vi "FPGA VI_Multiple Groups_Multiple Rates_Simulated_WithNoise_Example.vi"() -> ()   [LabVIEW 2019]
uses:
  <vilib>/rvi/DataTransferAndStorage/Container/XNode/niFpgaContainer.xnode
  <vilib>/Platform/TimedLoop/XDataNode/XDataNode.xnode
  <vilib>/Platform/TimedLoop/XDataNode/nitl_modes.ctl
  <vilib>/Platform/TimedLoop/XDataNode/XDNodeRunTimeDep.lvlib
  <vilib>/Platform/TimedLoop/XDataNode/wakeup.ctl
  <vilib>/Platform/TimedLoop/XDataNode/timing_clust.ctl
  <vilib>/rvi/FIFO/Fifo_Resource/niFpgaFifoEmulationRefIn.vi
  Types/Injection.Core.Internal.Settings.ctl
  <vilib>/rvi/LocalResourceManager/LocalResourceManager.xnode
  <vilib>/rvi/DataTransferAndStorage/Container/Common/niFpgaContainerGetUniqueNameForEmu.vi
  <vilib>/rvi/DataTransferAndStorage/Container/Common/niFpgaContainerSetEmuInfo.vi
  <vilib>/rvi/eio/common/nirviEmuReportErrorAndStop.vi
  <vilib>/rvi/Memory/Memory_Emulation/nirvimemoryFastEmulation.vi
  <vilib>/rvi/Memory/Memory_Emulation/nirvimemoryEmulation.vi
  Types/Injection.Mux.State.ctl
  <vilib>/rvi/interface/RandomDataEmulation/nirviRandomDataFpgaReadWriteTemplate.vi
  Types/Injection.Timing.ctl
  Types/Injection.Core.Settings.ctl
  Types/Injection.Global.Settings.ctl
panel:
  out "Intermediate FIFO Write Timeout 2":bool
  in  "Settings.Global.DUT1":T1={"Enable?"=FALSE, "Initial Voltage Threshold"=12.0, "Event Dwell Limit"=2000, "Voltage Gain"=1.0, "Current Gain"=1.0, "Filter Samples"=5, "Pretrigger Samples"=5, "Active Edge"=TRUE}
  in  "Settings.Index0.DUT1.Injector0":T2
  in  "Settings.Index1.DUT1.Injector1":T2
  in  "Settings.Index2.DUT1.Injector2":T2
  in  "Settings.Index3.DUT1.Injector3":T2
  out "Acqusition Loop Ticks 2":u32
  in  "Settings.Timing.DUT1":T3={"Injection Sample Period (Ticks)"=80}
  in  "Settings.Global.DUT2":T1={"Enable?"=FALSE, "Initial Voltage Threshold"=12.0, "Event Dwell Limit"=2000, "Voltage Gain"=1.0, "Current Gain"=1.0, "Filter Samples"=5, "Pretrigger Samples"=5, "Active Edge"=TRUE}
  in  "Settings.Index6.DUT2.Injector2":T2
  in  "Settings.Index7.DUT2.Injector3":T2
  out "Intermediate FIFO Write Timeout":bool
  in  "Settings.Index4.DUT2.Injector0":T2
  in  "Settings.Index5.DUT2.Injector1":T2
  in  "Settings.Timing.DUT2":T3={"Injection Sample Period (Ticks)"=320}
  out "Acqusition Loop Ticks":u32
  in  "Settings.DMA":cluster{"# of Injectors":u8}={"# of Injectors"=8}
  out "Host DMA Out?":bool
  out "Intermediate Time Out?":bool
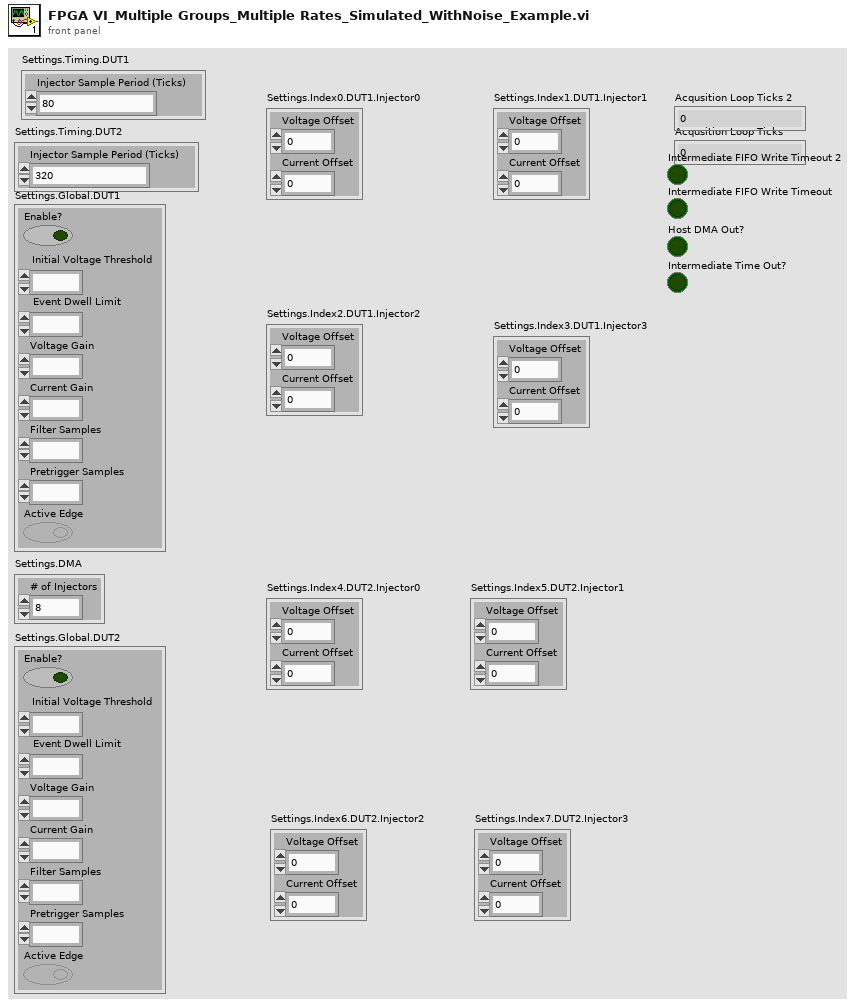
[diagram p1: front panel]
types:
  T1 = typedef "Injection.Global.Settings.ctl" = cluster{"Enable?":bool, "Initial Voltage Threshold":fxp<+/-,32,8>, "Event Dwell Limit":u16, "Voltage Gain":fxp<+/-,32,8>, "Current Gain":fxp<+/-,32,8>, "Filter Samples":u8, "Pretrigger Samples":u8, "Active Edge":bool}
  T2 = typedef "Injection.Core.Settings.ctl" = cluster{"Voltage Offset":fxp<+/-,32,8>, "Current Offset":fxp<+/-,32,8>}
  T3 = typedef "Injection.Timing.ctl" = cluster{"Injection Sample Period (Ticks)":u32}
  T4 = cluster{"Data.Samples":u32, "Injection.Period":u32, "Injector.Index":u8, "Iteration":u32}
  T5 = typedef "Injection.Mux.State.ctl" = enum8{"Wait on Transfer", "Transfer Injector Index", "Transfer # of Samples", "Transfer Injection Period", "Transfer Data Samples"}
  T6 = typedef "Injection.Core.Internal.Settings.ctl" = cluster{"Data Buffer FIFO":refnum<k21>, "Capture Complete Trigger FIFO":refnum<k21>}
  T7 = typedef "XDNodeRunTimeDep.lvlib/timing_clust.ctl" = cluster{"Expected End [f-1]":u64, "Actual End [f-1]":u64, "Finished Late? [f-1]":bool, "Expected End [i-1]":u64, "Actual End [i-1]":u64, "Finished Late? [i-1]":bool, "Expected Start [i]":u64, "Actual Start [i]":u64, "Expected Start [f]":u64, "Actual Start [f]":u64, "Source Name":string, "Structure Name":string, "Period":i64, "Deadline":i64, "Offset":i64, "Start":i64, "Priority":i32, "Timeout":i32, "Mode":T8, "Wakeup Reason":T9, "Error":errorcluster, "Source Type":string, "Secondary Source Type":string, "Global End Time":u64, "Global Start Time":u64, "Frame Duration":u64, "Iteration Duration":u64, "Assigned CPU":i32, "I/O Scan Engine Mode":u32}
  T8 = typedef "XDNodeRunTimeDep.lvlib/nitl_modes.ctl" = enum32{"No Change", "Process missed periods, maintain original phase", "Discard missed periods, maintain original phase", "Process missed periods, ignore original phase", "Discard missed periods, ignore original phase"}
  T9 = typedef "XDNodeRunTimeDep.lvlib/wakeup.ctl" = enum32{"Normal", "Aborted", "Asynchronous wakeup", "Timing source error", "Timed loop error", "Timeout"}
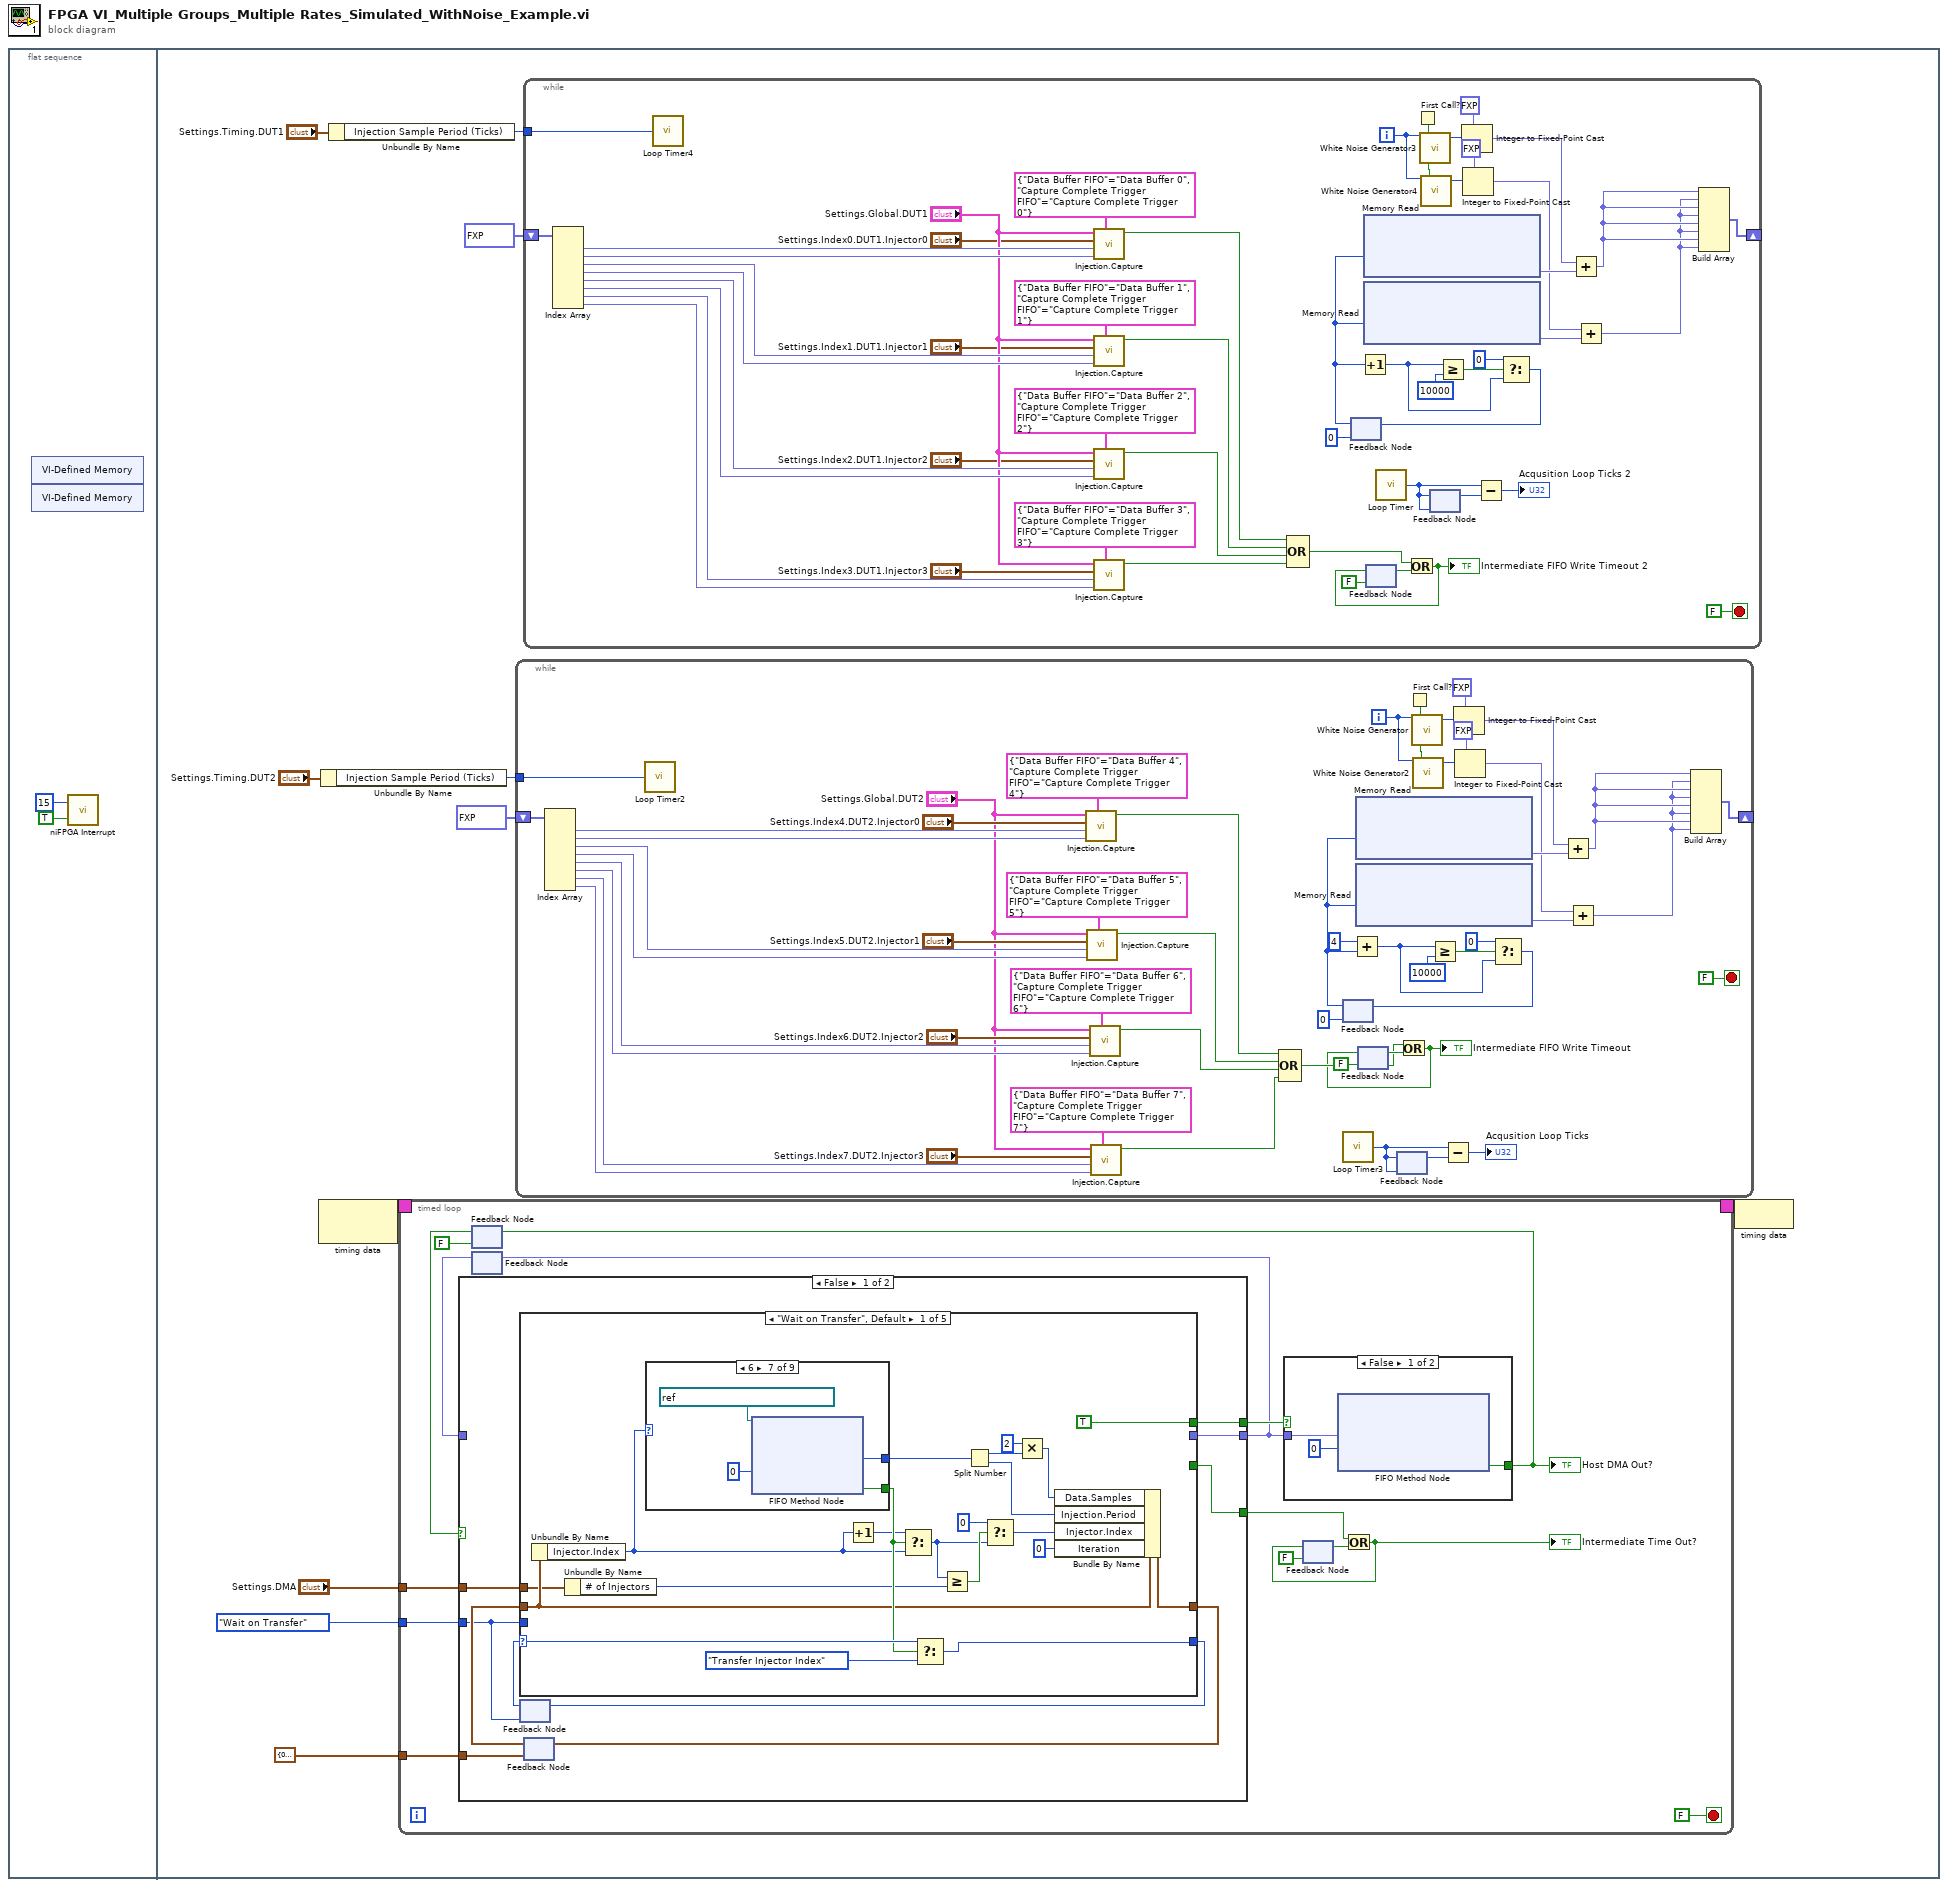
[diagram p0: block diagram]
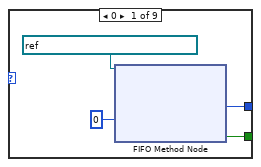
[diagram p2: hidden frame]
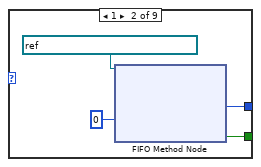
[diagram p3: hidden frame]
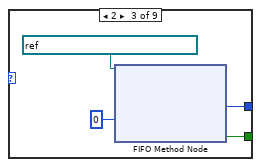
[diagram p4: hidden frame]
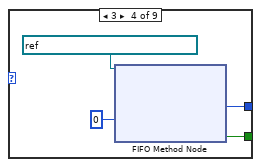
[diagram p5: hidden frame]
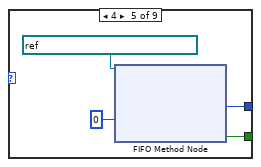
[diagram p6: hidden frame]
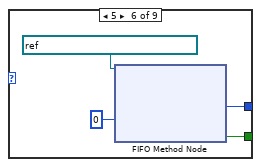
[diagram p7: hidden frame]
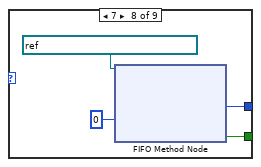
[diagram p8: hidden frame]
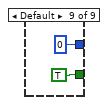
[diagram p9: hidden frame]
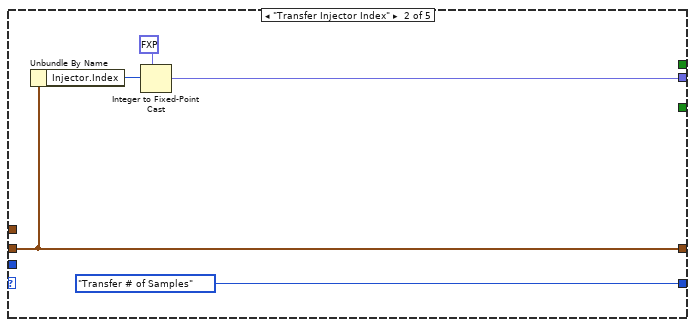
[diagram p10: hidden frame]
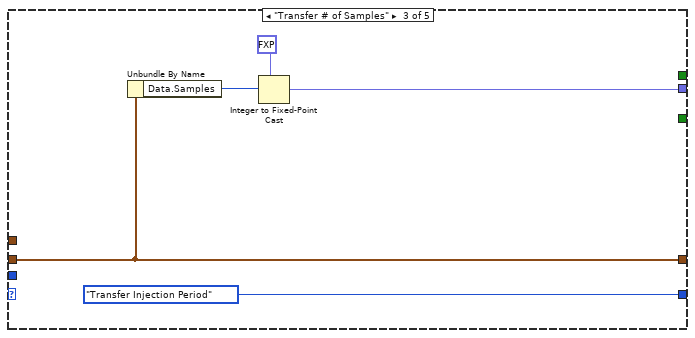
[diagram p11: hidden frame]
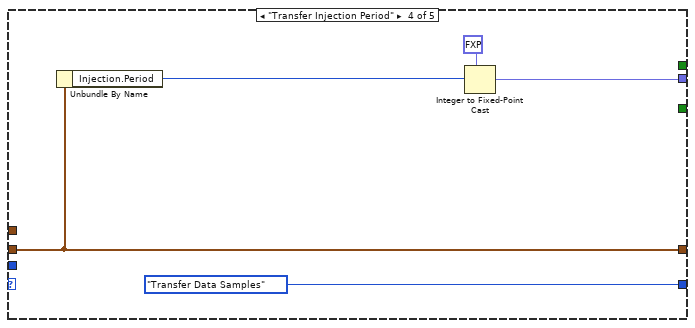
[diagram p12: hidden frame]
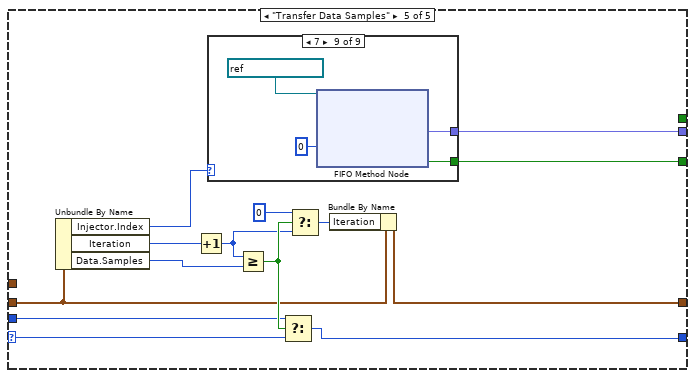
[diagram p13: hidden frame]
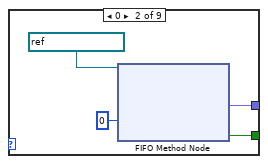
[diagram p15: hidden frame]
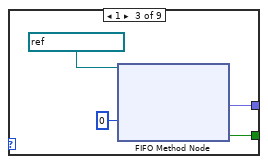
[diagram p16: hidden frame]
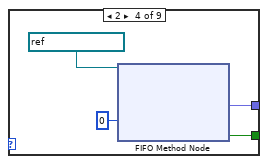
[diagram p17: hidden frame]
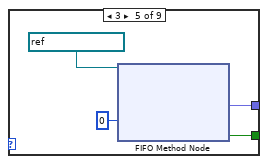
[diagram p18: hidden frame]
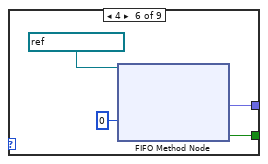
[diagram p19: hidden frame]
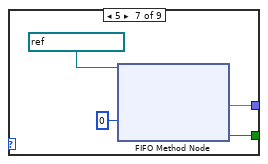
[diagram p20: hidden frame]
diagram:
  n1 = flat-sequence {
    frame #0 {
      n2 = xnode "VI-Defined Memory"() -> ()  [unwired: 1 out]
      n3 = xnode "VI-Defined Memory"() -> ()  [unwired: 1 out]
      n4 = call <vilib>:"niFPGA Interrupt.vi"("Wait Until Cleared (F)"=TRUE, "IRQ Number (0)"=u8 15) -> ()  [unwired: 1 in]
    }
    frame #1 {
      n5 = node-c288() -> (w13:T7)  [unwired: 1 in]
      n6 = Unbundle By Name("Settings.Timing.DUT2") -> ("Injection Sample Period (Ticks)"=w6:u32)
      n7 = Unbundle By Name("Settings.Timing.DUT1") -> ("Injection Sample Period (Ticks)"=w5:u32)
      n8 = timed-loop {
        timing: w13 -> [_]
        timing-out: [_] -> w12
        tunnel: "Settings.DMA" -> [w68]
        tunnel: Injection.Mux.State."Wait on Transfer" -> [w67]
        tunnel: T4 {"Data.Samples"=0, "Injection.Period"=0, "Injector.Index"=0, "Iteration"=0} ("Local.Data") -> [w66]
        stop <- FALSE stop-if-true
        n9 = feedback #1(FALSE ("Timed Out?")) -> (w76:bool)
        n10 = feedback #2() -> (w73:fxp<+/-,32,8>)  [unwired: 1 in]
        n11 = case shown="False" w76 {
          tunnel: [w88 w206] -> w74
          tunnel: [w87 w205] -> w78
          tunnel: w67 -> [w81 _]
          tunnel: [w86 w205] -> w69
          tunnel: w68 -> [w85 _]
          tunnel: w66 -> [w82 _]
          tunnel: w73 -> [_ w206]
          frame False {
            n12 = feedback #3(w81) -> (w80:T5)
            n13 = feedback #4(w82) -> (w83:T4)
            n14 = case shown="\"Wait on Transfer\", Default" w80 {
              selector: w80 -> [w109 _ _ _ w166]
              tunnel: w83 -> [w100 w147 w151 w155 w164]
              tunnel: [w108 w147 w151 w155 w163] -> w84
              tunnel: [w107 Injection.Mux.State."Transfer # of Samples" Injection.Mux.State."Transfer Injection Period" Injection.Mux.State."Transfer Data Samples" w165] -> w79
              tunnel: [_ w146 w150 w157 w162] -> w88
              tunnel: [TRUE _ _ _ _] -> w87
              tunnel: w81 -> [_ _ _ _ w159]
              tunnel: [_ _ _ _ w161] -> w86
              tunnel: w85 -> [w97 _ _ _ _]
              frame "Wait on Transfer", Default {
                n15 = Unbundle By Name(w100) -> ("Injector.Index"=w99:u8)
                n16 = Unbundle By Name(w97) -> ("# of Injectors"=w96:u8)
                n17 = case shown="6" w99 {
                  tunnel: [w112 w116 w120 w124 w128 w132 w136 w140 u64 0 ("Element")] -> w95
                  tunnel: [w111 w115 w119 w123 w127 w131 w135 w139 TRUE ("Timed Out?")] -> w105
                  frame 0 {
                    n18 = xnode ("FIFO Method Node")("Timeout"=0, "FIFO In"=refnum<k21> "Capture Complete Trigger 0") -> ("Element"=w112:u64, "Timed Out?"=w111:bool)  [unwired: 1 out]
                  }
                  frame 1 {
                    n19 = xnode ("FIFO Method Node")("Timeout"=0, "FIFO In"=refnum<k21> "Capture Complete Trigger 1") -> ("Element"=w116:u64, "Timed Out?"=w115:bool)  [unwired: 1 out]
                  }
                  frame 2 {
                    n20 = xnode ("FIFO Method Node")("Timeout"=0, "FIFO In"=refnum<k21> "Capture Complete Trigger 2") -> ("Element"=w120:u64, "Timed Out?"=w119:bool)  [unwired: 1 out]
                  }
                  frame 3 {
                    n21 = xnode ("FIFO Method Node")("Timeout"=0, "FIFO In"=refnum<k21> "Capture Complete Trigger 3") -> ("Element"=w124:u64, "Timed Out?"=w123:bool)  [unwired: 1 out]
                  }
                  frame 4 {
                    n22 = xnode ("FIFO Method Node")("Timeout"=0, "FIFO In"=refnum<k21> "Capture Complete Trigger 4") -> ("Element"=w128:u64, "Timed Out?"=w127:bool)  [unwired: 1 out]
                  }
                  frame 5 {
                    n23 = xnode ("FIFO Method Node")("Timeout"=0, "FIFO In"=refnum<k21> "Capture Complete Trigger 5") -> ("Element"=w132:u64, "Timed Out?"=w131:bool)  [unwired: 1 out]
                  }
                  frame 6 {
                    n24 = xnode ("FIFO Method Node")("Timeout"=0, "FIFO In"=refnum<k21> "Capture Complete Trigger 6") -> ("Element"=w136:u64, "Timed Out?"=w135:bool)  [unwired: 1 out]
                  }
                  frame 7 {
                    n25 = xnode ("FIFO Method Node")("Timeout"=0, "FIFO In"=refnum<k21> "Capture Complete Trigger 7") -> ("Element"=w140:u64, "Timed Out?"=w139:bool)  [unwired: 1 out]
                  }
                  frame Default {
                  }
                }
                n26 = Increment(x=w99) -> (x+1=w104:u8)
                n27 = Select(t=w104, s=w105, f=w99) -> (s? t:f=w102:u8)
                n28 = Select(t=w109, s=w105, f=Injection.Mux.State."Transfer Injector Index") -> (s? t:f=w107:T5)
                n29 = Greater Or Equal?(x=w102, y=w96) -> (x >= y?=w103:bool)
                n30 = Split Number(x=w95) -> (hi(x)=w94:u32, lo(x)=w93:u32)
                n31 = Select(t=u8 0, s=w103, f=w102) -> (s? t:f=w98:u8)
                n32 = Multiply(x=u32 2, y=w94) -> (x*y=w91:u32)
                n33 = Bundle By Name(cluster=w100, "Data.Samples"=w91, "Injection.Period"=w93, "Injector.Index"=w98, "Iteration"=u32 0) -> (w108:T4)
              }
              frame "Transfer Injector Index" {
                n34 = Unbundle By Name(w147) -> ("Injector.Index"=w148:u8)
                n35 = Integer to Fixed-Point Cast(fixed-point type=fxp<+/-,32,8> 0.0, integer=w148) -> (fixed-point=w146:fxp<+/-,32,8>)
              }
              frame "Transfer # of Samples" {
                n36 = Unbundle By Name(w151) -> ("Data.Samples"=w152:u32)
                n37 = Integer to Fixed-Point Cast(fixed-point type=fxp<+/-,32,8> 0.0, integer=w152) -> (fixed-point=w150:fxp<+/-,32,8>)
              }
              frame "Transfer Injection Period" {
                n38 = Unbundle By Name(w155) -> ("Injection.Period"=w156:u32)
                n39 = Integer to Fixed-Point Cast(fixed-point type=fxp<+/-,32,8> 0.0, integer=w156) -> (fixed-point=w157:fxp<+/-,32,8>)
              }
              frame "Transfer Data Samples" {
                n40 = Unbundle By Name(w164) -> ("Injector.Index"=w172:u8, "Iteration"=w167:u32, "Data.Samples"=w160:u32)
                n41 = Increment(x=w167) -> (x+1=w169:u32)
                n42 = case shown="7" w172 {
                  tunnel: [_ w175 w179 w183 w187 w191 w195 w199 w203] -> w162
                  tunnel: [_ w174 w178 w182 w186 w190 w194 w198 w202] -> w161
                  frame Default {
                  }
                  frame 0 {
                    n43 = xnode ("FIFO Method Node")("Timeout"=0, "FIFO In"=refnum<k21> "Data Buffer 0" ("Voltage FIFO")) -> ("Element"=w175:fxp<+/-,32,8>, "Timed Out?"=w174:bool)  [unwired: 1 out]
                  }
                  frame 1 {
                    n44 = xnode ("FIFO Method Node")("Timeout"=0, "FIFO In"=refnum<k21> "Data Buffer 1" ("Voltage FIFO")) -> ("Element"=w179:fxp<+/-,32,8>, "Timed Out?"=w178:bool)  [unwired: 1 out]
                  }
                  frame 2 {
                    n45 = xnode ("FIFO Method Node")("Timeout"=0, "FIFO In"=refnum<k21> "Data Buffer 2" ("Voltage FIFO")) -> ("Element"=w183:fxp<+/-,32,8>, "Timed Out?"=w182:bool)  [unwired: 1 out]
                  }
                  frame 3 {
                    n46 = xnode ("FIFO Method Node")("Timeout"=0, "FIFO In"=refnum<k21> "Data Buffer 3" ("Voltage FIFO")) -> ("Element"=w187:fxp<+/-,32,8>, "Timed Out?"=w186:bool)  [unwired: 1 out]
                  }
                  frame 4 {
                    n47 = xnode ("FIFO Method Node")("Timeout"=0, "FIFO In"=refnum<k21> "Data Buffer 4" ("Voltage FIFO")) -> ("Element"=w191:fxp<+/-,32,8>, "Timed Out?"=w190:bool)  [unwired: 1 out]
                  }
                  frame 5 {
                    n48 = xnode ("FIFO Method Node")("Timeout"=0, "FIFO In"=refnum<k21> "Data Buffer 5" ("Voltage FIFO")) -> ("Element"=w195:fxp<+/-,32,8>, "Timed Out?"=w194:bool)  [unwired: 1 out]
                  }
                  frame 6 {
                    n49 = xnode ("FIFO Method Node")("Timeout"=0, "FIFO In"=refnum<k21> "Data Buffer 6" ("Voltage FIFO")) -> ("Element"=w199:fxp<+/-,32,8>, "Timed Out?"=w198:bool)  [unwired: 1 out]
                  }
                  frame 7 {
                    n50 = xnode ("FIFO Method Node")("Timeout"=0, "FIFO In"=refnum<k21> "Data Buffer 7" ("Voltage FIFO")) -> ("Element"=w203:fxp<+/-,32,8>, "Timed Out?"=w202:bool)  [unwired: 1 out]
                  }
                }
                n51 = Greater Or Equal?(x=w169, y=w160) -> (x >= y?=w171:bool)
                n52 = Select(t=w159, s=w171, f=w166) -> (s? t:f=w165:T5)
                n53 = Select(t=u32 0, s=w171, f=w169) -> (s? t:f=w168:u32)
                n54 = Bundle By Name(cluster=w164, "Iteration"=w168) -> (w163:T4)
              }
            }
            n55 = feedback-in #3(w79) -> ()
            n56 = feedback-in #4(w84) -> ()
          }
          frame True {
            w205 = FALSE
          }
        }
        n57 = feedback-in #2(w74) -> ()
        n58 = case shown="False" w78 {
          tunnel: w74 -> [w208 _]
          tunnel: [w207 FALSE ("Timed Out?")] -> w77
          frame False {
            n59 = xnode ("FIFO Method Node")("Element"=w208, "Timeout"=0) -> ("Timed Out?"=w207:bool)  [unwired: 1 in, 1 out]
          }
          frame True {
          }
        }
        "Host DMA Out?" <- w77
        n60 = feedback-in #1(w77) -> ()
        n61 = feedback #5(FALSE ("Timed Out?")) -> (w71:bool)
        n62 = Or(x=w69, y=w71) -> (x .or. y?=w70:bool)
        "Intermediate Time Out?" <- w70
        n63 = feedback-in #5(w70) -> ()
      }
      n64 = while {
        shift-right: [w238] -> _
        shift-left: fxp<+/-,24,5>[] [0.0, 0.0, 0.0, 0.0, 0.0, 0.0, 0.0, 0.0] -> [w260]
        tunnel: w6 -> [w249]
        i -> [w233]
        stop <- FALSE stop-if-true
        n65 = Index Array(array=w260) -> (element #1=w263:fxp<+/-,24,5>, element #2=w264:fxp<+/-,24,5>, element #3=w261:fxp<+/-,24,5>, element #4=w262:fxp<+/-,24,5>, element #5=w224:fxp<+/-,24,5>, element #6=w223:fxp<+/-,24,5>, element #7=w221:fxp<+/-,24,5>, element #8=w222:fxp<+/-,24,5>)  [unwired: 8 in]
        n66 = call "Loop Timer2"("Count(Ticks)"=w249) -> ()  [unwired: 1 out]
        n67 = call "Injection.Capture.vi"("FIFOs"=T6 {"Data Buffer FIFO"="Data Buffer 4", "Capture Complete Trigger FIFO"="Capture Complete Trigger 4"} ("InjectorCore.Settings"), "Current (PreScaled)"=w264, "Voltage (PreScaled)"=w263, "Settings.Index<#>.<Group>.<UserName>"="Settings.Index4.DUT2.Injector0", "Settings.Global.<Group>"="Settings.Global.DUT2") -> ("Intermediate FIFO Timeout?"=w266:bool)  [unwired: 4 in, 2 out]
        n68 = call "Injection.Capture.vi"("FIFOs"=T6 {"Data Buffer FIFO"="Data Buffer 5", "Capture Complete Trigger FIFO"="Capture Complete Trigger 5"} ("InjectorCore.Settings"), "Current (PreScaled)"=w262, "Voltage (PreScaled)"=w261, "Settings.Index<#>.<Group>.<UserName>"="Settings.Index5.DUT2.Injector1", "Settings.Global.<Group>"="Settings.Global.DUT2") -> ("Intermediate FIFO Timeout?"=w265:bool)  [unwired: 4 in, 2 out]
        n69 = call "Injection.Capture.vi"("FIFOs"=T6 {"Data Buffer FIFO"="Data Buffer 6", "Capture Complete Trigger FIFO"="Capture Complete Trigger 6"} ("InjectorCore.Settings"), "Current (PreScaled)"=w223, "Voltage (PreScaled)"=w224, "Settings.Index<#>.<Group>.<UserName>"="Settings.Index6.DUT2.Injector2", "Settings.Global.<Group>"="Settings.Global.DUT2") -> ("Intermediate FIFO Timeout?"=w219:bool)  [unwired: 4 in, 2 out]
        n70 = call "Injection.Capture.vi"("FIFOs"=T6 {"Data Buffer FIFO"="Data Buffer 7", "Capture Complete Trigger FIFO"="Capture Complete Trigger 7"} ("InjectorCore.Settings"), "Current (PreScaled)"=w222, "Voltage (PreScaled)"=w221, "Settings.Index<#>.<Group>.<UserName>"="Settings.Index7.DUT2.Injector3", "Settings.Global.<Group>"="Settings.Global.DUT2") -> ("Intermediate FIFO Timeout?"=w218:bool)  [unwired: 4 in, 2 out]
        n71 = Compound Arithmetic op=OR(w266, w265, w219, w218) -> (w254:bool)
        n72 = feedback #6(u32 0 ("Address")) -> (w245:u32)
        n73 = call "Loop Timer3"() -> ("Tick Count(Ticks)"=w250:u32)  [unwired: 1 in]
        n74 = Add(x=u32 4, y=w245) -> (x+y=w241:u32)
        n75 = xnode ("Memory Read")("Address"=w245) -> ("Data"=w246:fxp<+/-,24,5>)  [unwired: 1 in, 1 out]
        n76 = xnode ("Memory Read")("Address"=w245) -> ("Data"=w230:fxp<+/-,24,5>)  [unwired: 1 in, 1 out]
        n77 = feedback #7(FALSE ("Timed Out?")) -> (w255:bool)
        n78 = feedback-in #8(w250) -> ()
        n79 = feedback #8(w250) -> (w252:u32)
        n80 = Or(x=w254, y=w255) -> (x .or. y?=w253:bool)
        "Intermediate FIFO Write Timeout" <- w253
        n81 = feedback-in #7(w253) -> ()
        n82 = First Call?() -> (First Call?: T/F=w229:bool)
        n83 = call "White Noise Generator"("seed"=w233, "reset"=w229) -> ("white noise out"=w237:i16)  [unwired: 13 in]
        n84 = call "White Noise Generator2"("seed"=w233, "reset"=w229) -> ("white noise out"=w234:i16)  [unwired: 13 in]
        n85 = Greater Or Equal?(x=w241, y=u32 10000) -> (x >= y?=w240:bool)
        n86 = Subtract(x=w250, y=w252) -> (x-y=→"Acqusition Loop Ticks":u32)
        n87 = Integer to Fixed-Point Cast(fixed-point type=fxp<+/-,24,5> 0.0, integer=w237) -> (fixed-point=w232:fxp<+/-,24,5>)
        n88 = Integer to Fixed-Point Cast(fixed-point type=fxp<+/-,24,5> 0.0, integer=w234) -> (fixed-point=w231:fxp<+/-,24,5>)
        n89 = Select(t=u32 0, s=w240, f=w241) -> (s? t:f=w243:u32)
        n90 = feedback-in #6(w243) -> ()
        n91 = Add(x=w232, y=w246) -> (x+y=w217:fxp<+/-,24,5>)
        n92 = Add(x=w231, y=w230) -> (x+y=w216:fxp<+/-,24,5>)
        n93 = Build Array(w217, w216, w217, w216, w217, w216, w217, w216) -> (w238:fxp<+/-,24,5>[])
      }
      n94 = while {
        shift-right: [w25] -> _
        shift-left: fxp<+/-,24,5>[] [0.0, 0.0, 0.0, 0.0, 0.0, 0.0, 0.0, 0.0] -> [w51]
        tunnel: w5 -> [w37]
        i -> [w20]
        stop <- FALSE stop-if-true
        n95 = Index Array(array=w51) -> (element #1=w58:fxp<+/-,24,5>, element #2=w59:fxp<+/-,24,5>, element #3=w56:fxp<+/-,24,5>, element #4=w57:fxp<+/-,24,5>, element #5=w54:fxp<+/-,24,5>, element #6=w55:fxp<+/-,24,5>, element #7=w52:fxp<+/-,24,5>, element #8=w53:fxp<+/-,24,5>)  [unwired: 8 in]
        n96 = call "Loop Timer4"("Count(Ticks)"=w37) -> ()  [unwired: 1 out]
        n97 = call "Injection.Capture.vi"("FIFOs"=T6 {"Data Buffer FIFO"="Data Buffer 0", "Capture Complete Trigger FIFO"="Capture Complete Trigger 0"} ("InjectorCore.Settings"), "Current (PreScaled)"=w59, "Voltage (PreScaled)"=w58, "Settings.Index<#>.<Group>.<UserName>"="Settings.Index0.DUT1.Injector0", "Settings.Global.<Group>"="Settings.Global.DUT1") -> ("Intermediate FIFO Timeout?"=w64:bool)  [unwired: 4 in, 2 out]
        n98 = call "Injection.Capture.vi"("FIFOs"=T6 {"Data Buffer FIFO"="Data Buffer 1", "Capture Complete Trigger FIFO"="Capture Complete Trigger 1"} ("InjectorCore.Settings"), "Current (PreScaled)"=w57, "Voltage (PreScaled)"=w56, "Settings.Index<#>.<Group>.<UserName>"="Settings.Index1.DUT1.Injector1", "Settings.Global.<Group>"="Settings.Global.DUT1") -> ("Intermediate FIFO Timeout?"=w63:bool)  [unwired: 4 in, 2 out]
        n99 = call "Injection.Capture.vi"("FIFOs"=T6 {"Data Buffer FIFO"="Data Buffer 2", "Capture Complete Trigger FIFO"="Capture Complete Trigger 2"} ("InjectorCore.Settings"), "Current (PreScaled)"=w55, "Voltage (PreScaled)"=w54, "Settings.Index<#>.<Group>.<UserName>"="Settings.Index2.DUT1.Injector2", "Settings.Global.<Group>"="Settings.Global.DUT1") -> ("Intermediate FIFO Timeout?"=w62:bool)  [unwired: 4 in, 2 out]
        n100 = call "Injection.Capture.vi"("FIFOs"=T6 {"Data Buffer FIFO"="Data Buffer 3", "Capture Complete Trigger FIFO"="Capture Complete Trigger 3"} ("InjectorCore.Settings"), "Current (PreScaled)"=w53, "Voltage (PreScaled)"=w52, "Settings.Index<#>.<Group>.<UserName>"="Settings.Index3.DUT1.Injector3", "Settings.Global.<Group>"="Settings.Global.DUT1") -> ("Intermediate FIFO Timeout?"=w61:bool)  [unwired: 4 in, 2 out]
        n101 = Compound Arithmetic op=OR(w64, w63, w62, w61) -> (w42:bool)
        n102 = feedback #9(u32 0 ("Address")) -> (w32:u32)
        n103 = Increment(x=w32) -> (x+1=w28:u32)
        n104 = xnode ("Memory Read")("Address"=w32) -> ("Data"=w33:fxp<+/-,24,5>)  [unwired: 1 in, 1 out]
        n105 = xnode ("Memory Read")("Address"=w32) -> ("Data"=w17:fxp<+/-,24,5>)  [unwired: 1 in, 1 out]
        n106 = feedback #10(FALSE ("Timed Out?")) -> (w43:bool)
        n107 = call "Loop Timer"() -> ("Tick Count(Ticks)"=w38:u32)  [unwired: 1 in]
        n108 = Or(x=w42, y=w43) -> (x .or. y?=w41:bool)
        "Intermediate FIFO Write Timeout 2" <- w41
        n109 = feedback-in #10(w41) -> ()
        n110 = First Call?() -> (First Call?: T/F=w16:bool)
        n111 = call "White Noise Generator3"("seed"=w20, "reset"=w16) -> ("white noise out"=w24:i16)  [unwired: 13 in]
        n112 = call "White Noise Generator4"("seed"=w20, "reset"=w16) -> ("white noise out"=w21:i16)  [unwired: 13 in]
        n113 = feedback-in #11(w38) -> ()
        n114 = feedback #11(w38) -> (w40:u32)
        n115 = Greater Or Equal?(x=w28, y=u32 10000) -> (x >= y?=w27:bool)
        n116 = Integer to Fixed-Point Cast(fixed-point type=fxp<+/-,24,5> 0.0, integer=w24) -> (fixed-point=w19:fxp<+/-,24,5>)
        n117 = Integer to Fixed-Point Cast(fixed-point type=fxp<+/-,24,5> 0.0, integer=w21) -> (fixed-point=w18:fxp<+/-,24,5>)
        n118 = Subtract(x=w38, y=w40) -> (x-y=→"Acqusition Loop Ticks 2":u32)
        n119 = Select(t=u32 0, s=w27, f=w28) -> (s? t:f=w30:u32)
        n120 = feedback-in #9(w30) -> ()
        n121 = Add(x=w19, y=w33) -> (x+y=w15:fxp<+/-,24,5>)
        n122 = Add(x=w18, y=w17) -> (x+y=w14:fxp<+/-,24,5>)
        n123 = Build Array(w15, w14, w15, w14, w15, w14, w15, w14) -> (w25:fxp<+/-,24,5>[])
      }
      n124 = node-c288(w12) -> ()
    }
  }
